vi "TestVIDates.vi"() -> ()   [LabVIEW 2017]
uses:
  <vilib>/Utility/config.llb/Read Key (String).vi
  <vilib>/Utility/config.llb/Write Key (String).vi
  <vilib>/Utility/config.llb/NI_LVConfig.lvlib
panel:
  out "last mod":timestamp
  out "Generate":bool
  out "array":string[][](array[string])
  out "standard error":string
  out "standard output":string
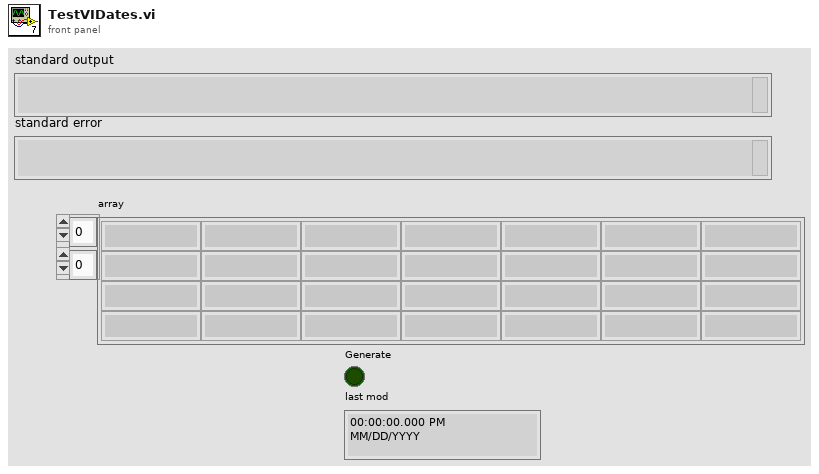
[diagram p1: front panel]
types:
  T1 = typedef "NI_LVConfig.lvlib/Config Data RefNum.ctl" = refnum<k1>
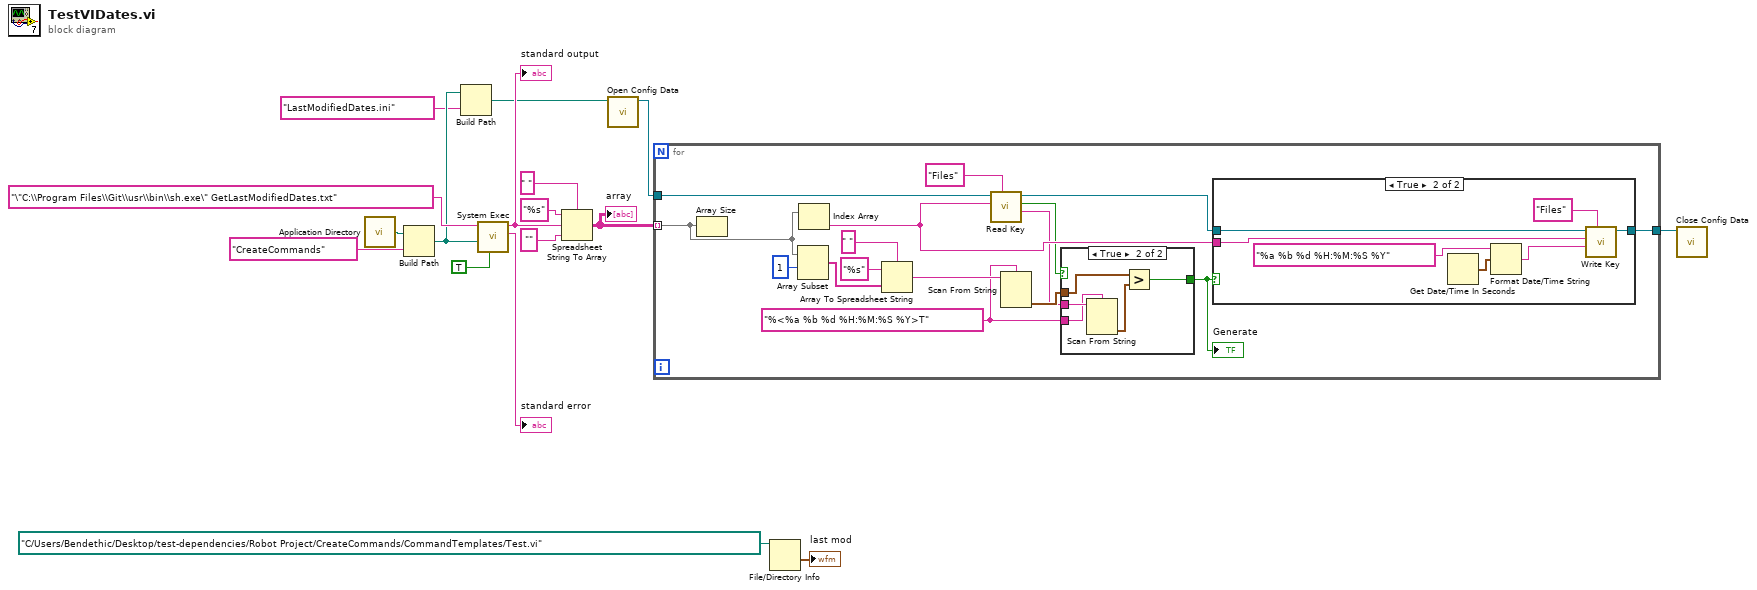
[diagram p0: block diagram]
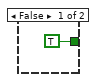
[diagram p3: hidden frame]
diagram:
  n1 = call <vilib>:"Application Directory.vi"() -> ("Application Directory"=w16:path)
  n2 = Build Path(base path=w16, name or relative path="CreateCommands") -> (appended path=w7:path)
  n3 = Build Path(base path=w7, name or relative path="LastModifiedDates.ini") -> (appended path=w5:path)
  n4 = call <vilib>:"System Exec.vi"("run minimized? (F)"=TRUE, "working directory"=w7, "command line"="\"C:\\Program Files\\Git\\usr\\bin\\sh.exe\" GetLastModifiedDates.txt") -> ("standard error"=→"standard error":string, "standard output"=w11:string)  [unwired: 5 in, 2 out]
  "standard output" <- w11
  n5 = Spreadsheet String To Array(delimiter (Tab)=" ", format string="%s", spreadsheet string=w11, array type (2D Dbl)="" ("standard output")) -> (array=w8:string[][])
  "array" <- w8
  n6 = call <vilib>:"Open Config Data.vi"("configuration file path"=w5) -> ("refnum"=w4:T1)  [unwired: 8 in, 2 out]
  n7 = for {
    tunnel: w8 -> [w29] mode=indexing
    tunnel: w4 -> [w28]
    tunnel: [w22] -> w3
    w20 = "%<%a %b %d %H:%M:%S %Y>T" ("format string")
    n8 = Array Size(array=w29) -> ()  [unwired: 1 out]
    n9 = Array Subset(array=w29, index=1) -> (w32:string[])  [unwired: 1 in]
    n10 = Index Array(array=w29) -> (element=w23:string)  [unwired: 1 in]
    n11 = Array To Spreadsheet String(delimiter (Tab)=" ", array=w32, 3:"%s" ("format string")) -> (spreadsheet string=w30:string)
    n12 = call-poly <vilib>:"Read Key.vi"("section"="Files", "key"=w23, "refnum"=w28) -> ("value"=w21:string, "found?"=w19:bool, "refnum out"=w24:T1)  [unwired: 5 in, 1 out]
    n13 = Scan From String(format string=w20, input string=w30) -> (output 1=w26:timestamp)  [unwired: 3 in, 3 out]
    n14 = case shown="True" w19 {
      tunnel: [TRUE ("run minimized? (F)") w47] -> w25
      tunnel: w26 -> [_ w46]
      tunnel: w21 -> [_ w45]
      tunnel: w20 -> [_ w43]
      frame False {
      }
      frame True {
        n15 = Scan From String(format string=w43, input string=w45) -> (output 1=w44:timestamp)  [unwired: 3 in, 3 out]
        n16 = Greater?(x=w46, y=w44) -> (0:w47:bool)
      }
    }
    "Generate" <- w25
    n17 = case shown="True" w25 {
      tunnel: w24 -> [w34 w38]
      tunnel: w23 -> [_ w37]
      tunnel: [w34 w35] -> w22
      frame False {
      }
      frame True {
        n18 = Get Date/Time In Seconds() -> (seconds since 1Jan1904=w40:timestamp)
        n19 = Format Date/Time String(time format string (%c)="%a %b %d %H:%M:%S %Y", seconds (now)=w40) -> (date/time string=w39:string)  [unwired: 1 in]
        n20 = call-poly <vilib>:"Write Key.vi"("section"="Files", "value"=w39, "key"=w37, "refnum"=w38) -> ("refnum out"=w35:T1)  [unwired: 5 in, 2 out]
      }
    }
  }
  n21 = File/Directory Info(path=path "C:/Users/Bendethic/Desktop/test-dependencies/Robot Project/CreateCommands/CommandTemplates/Test.vi") -> (last mod=→"last mod":timestamp)  [unwired: 1 in, 6 out]
  n22 = call <vilib>:"Close Config Data.vi"("refnum"=w3) -> ()  [unwired: 9 in, 2 out]
